vi "SetParam.vi"(8 "error in (no error)":errorcluster caption="entrée d'erreur (pas d'erreur)", 10 "LabelBinarizer":T1={"neg_label"=0, "pos_label"=1, "sparse_output"=FALSE}, 11 "LabelBinarizer.lvclass":refnum<class "LabelBinarizer.lvclass">) -> (0 "error out":errorcluster caption="sortie d'erreur", 3 "LabelBinarizer.lvclass":refnum<class "LabelBinarizer.lvclass">)   [LabVIEW 2020, in "LabelBinarizer.lvclass"]
doc: "Set Parameters"
uses:
  LabelBinarizer.lvclass
  LabelBinarizer.lvclass/LabelBinarizer.ctl
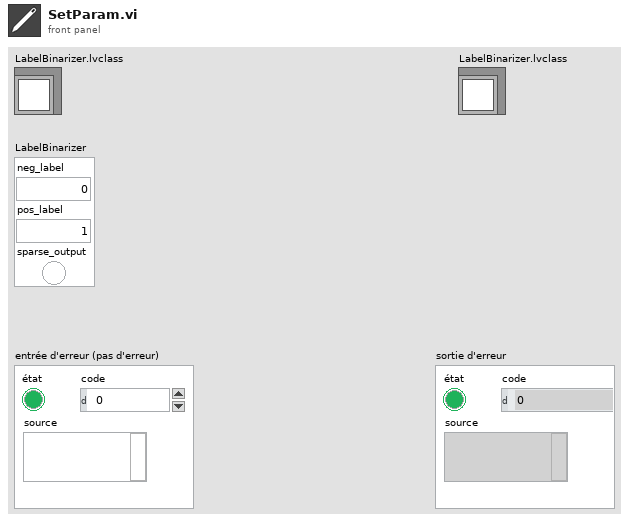
[diagram p1: front panel]
types:
  T1 = cluster{"neg_label":i32, "pos_label":i32, "sparse_output":bool}
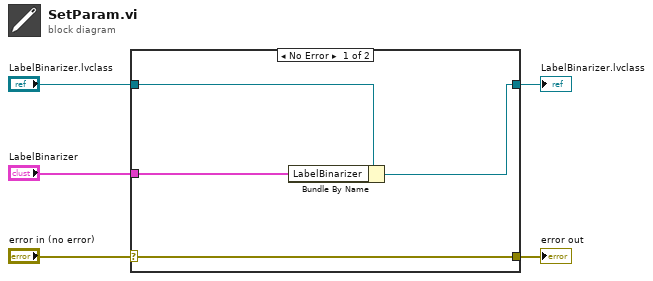
[diagram p0: block diagram]
diagram:
  n1 = case shown="No Error" "error in (no error)" {
    selector: "error in (no error)" -> [w9 w10]
    tunnel: [w9 w10] -> w4
    tunnel: [w7 w11] -> w2
    tunnel: "LabelBinarizer.lvclass" -> [w8 w11]
    tunnel: "LabelBinarizer" -> [w6 _]
    frame No Error {
      n2 = Bundle By Name(cluster=w8, "LabelBinarizer"=w6) -> (w7:refnum<class "LabelBinarizer.lvclass">)
    }
    frame Error {
    }
  }
  "error out" <- w4
  "LabelBinarizer.lvclass" <- w2
